vi "tiempo_real.vi"() -> ()   [LabVIEW 2011]
uses:
  <vilib>/Simulation/Scripting/Companion Diagram/SimConfigNode/SimParams.ctl
  <vilib>/Simulation/Scripting/Companion Diagram/SimConfigNode/_simSolvers.ctl
  <vilib>/Simulation/Implementation/Shared/SIMSCR Execution Mode.ctl
  <vilib>/Simulation/Param Hierarchy/Typedefs/SIMPH Param Control Actions.ctl
  <vilib>/Simulation/Implementation/Shared/NILVSim_FinalizeModel.vi
  <vilib>/Simulation/DiscreteLinear/Implementation/NILVSim Discrete Transfer Function Direct.llb/SIM Discrete Transfer Function Direct (SISO CD).vi
  <vilib>/Simulation/DiscreteLinear/Implementation/NILVSim Discrete ZOH.llb/SIM Discrete ZOH (scalar).vi
  <vilib>/Simulation/Nonlinear/Implementation/NILVSim Saturation.llb/SIM Saturation (scalar).vi
  <vilib>/Simulation/SignalDisplay/Implementation/NILVSim Time Waveform.llb/SIM Time Waveform (vector).vi
  <vilib>/Simulation/SignalDisplay/Implementation/NILVSim Time Waveform.llb/SIM Time Waveform (scalar).vi
  <vilib>/Simulation/Implementation/Shared/NILVSim_Manager.vi
  <vilib>/Simulation/Implementation/Shared/NILVSim_ParamChanged.vi
  <vilib>/Simulation/Utility/Implementation/NILVSim Get Time and IsAcceptedStep.vi
  <vilib>/addons/Control Design/_Model Construction/Model Creation.llb/Model Creation SubVI/cd_Create Transfer Function Model.vi
  <vilib>/addons/Control Design/_Utility/Model Viewer.llb/Model Viewer SubVI/cd_Draw Transfer Function Equation (TF).vi
  <vilib>/Simulation/Implementation/Shared/SIM Unbundle Sim Info.vi
  <vilib>/Simulation/Implementation/Shared/NILVSim_GetModelError.vi
  <vilib>/Simulation/Implementation/Shared/SIM Bundle Sim Info.vi
  <vilib>/Simulation/Implementation/Shared/NILVSim_Initialize.vi
  <vilib>/Simulation/Scripting/Companion Diagram/SimConfigNode/SimDog.xnode
  <vilib>/Simulation/Implementation/XNodeFramework/SimXNode/SimX.xnode
  <vilib>/addons/Control Design/_Model Construction/Model Typedefs.llb/CD Transfer Function Model (MIMO).ctl
  <vilib>/addons/Control Design/_Model Construction/Model Typedefs.llb/CD General Elements.ctl
  <vilib>/addons/Control Design/_Model Construction/Model Typedefs.llb/CD Transfer Function Model (SISO).ctl
  <vilib>/addons/Control Design/_Utility/NI_CD_Model Viewer.lvlib
  <vilib>/addons/Control Design/_Model Construction/NI_LinSys_Model Creation.lvlib
  <vilib>/addons/Control Design/_Model Construction/NI_LinSys_Model Typedefs.lvlib
  <vilib>/Simulation/Implementation/Shared/NI_SIM_Implementation.lvlib
panel:
  out "D(z)":picture
  out "?":waveform(dbl)(graph)={"t0"=timestamp(0 s since 1904-01-01), "dt"=1.0, "Y"=[0.0]}
  out "?":waveform(dbl)[](graph)=[{"t0"=timestamp(0 s since 1904-01-01), "dt"=1.0, "Y"=[4.028870584284064]}, {"t0"=timestamp(0 s since 1904-01-01), "dt"=1.0, "Y"=[4.030612244897959]}]
  in  "T":dbl=0.03
  in  "Set Point":dbl(slide)=4.030612244897959 scale=0.0..5.0
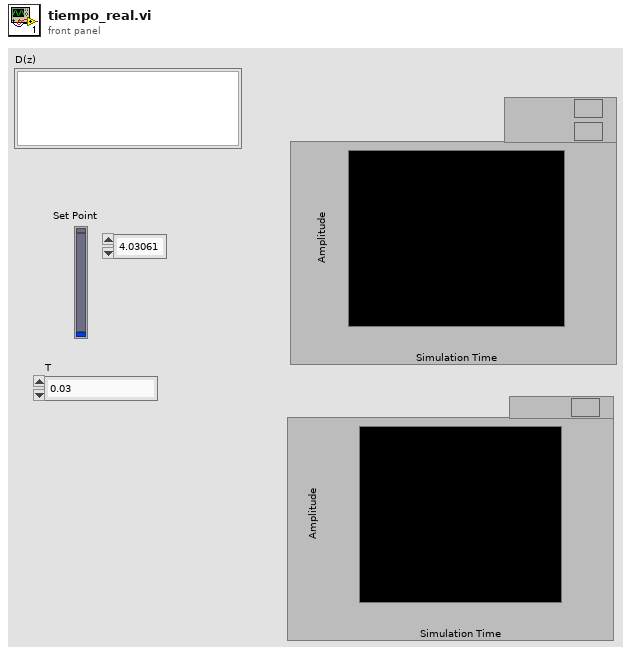
[diagram p1: front panel]
types:
  T1 = typedef "NI_LinSys_Model Typedefs.lvlib/CD Transfer Function Model (MIMO).ctl" = cluster{"properties":T2, "transfer function(s)":T3[][]}
  T2 = typedef "NI_LinSys_Model Typedefs.lvlib/CD General Elements.ctl" = cluster{"Model name":string, "Input names":string[], "Output names":string[], "Input Delays":dbl[], "Output Delays":dbl[], "Sampling Time":dbl, "Notes":string}
  T3 = typedef "NI_LinSys_Model Typedefs.lvlib/CD Transfer Function Model (SISO).ctl" = cluster{"Numerator":dbl[], "Denominator":dbl[], "delay":dbl}
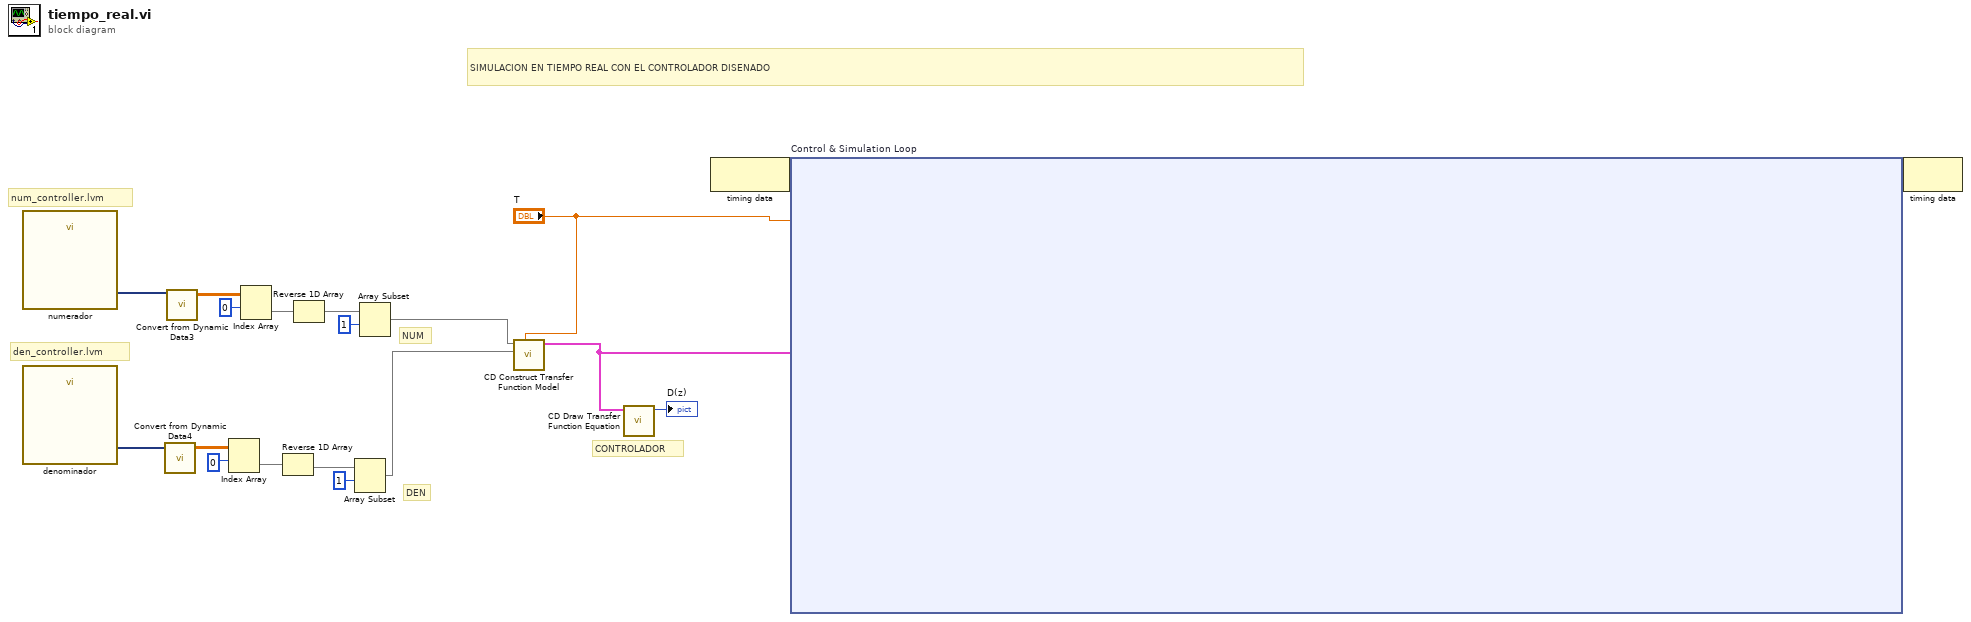
[diagram p0: block diagram]
diagram:
  # "SIMULACION EN TIEMPO REAL CON EL CONTROLADOR DISENADO"
  # "DEN"
  # "NUM"
  # "den_controller.lvm"
  # "num_controller.lvm"
  # "CONTROLADOR"
  n1 = call "numerador"() -> ("Signals"=w4:dynamicdata)  [unwired: 6 in, 5 out]
  n2 = call "denominador"() -> ("Signals"=w3:dynamicdata)  [unwired: 6 in, 5 out]
  n3 = call "Convert from Dynamic Data4"("Dynamic Data Type"=w3) -> ("Array"=w6:dbl[][])  [unwired: 3 in]
  n4 = call "Convert from Dynamic Data3"("Dynamic Data Type"=w4) -> ("Array"=w13:dbl[][])  [unwired: 3 in]
  n5 = Index Array(array=w6, index (row)=0) -> (element=w7:dbl[])  [unwired: 1 in]
  n6 = Index Array(array=w13, index (row)=0) -> (element=w12:dbl[])  [unwired: 1 in]
  n7 = Reverse 1D Array(array=w7) -> (reversed array=w8:dbl[])
  n8 = Reverse 1D Array(array=w12) -> (reversed array=w11:dbl[])
  n9 = Array Subset(array=w8, index=1) -> (w1:dbl[])  [unwired: 1 in]
  n10 = Array Subset(array=w11, index=1) -> (w2:dbl[])  [unwired: 1 in]
  n11 = call-poly <vilib>:"CD Construct Transfer Function Model.vi"("Sampling Time (s)"="T", "Denominator"=w1, "Numerator"=w2) -> ("Transfer Function Model"=w16:T1)  [unwired: 7 in, 1 out]
  n12 = call-poly <vilib>:"CD Draw Transfer Function Equation.vi"("Transfer Function Model"=w16) -> ("Equation"=→"D(z)":picture)  [unwired: 8 in, 2 out]
  n13 = node-c288() -> (w19:variant)  [unwired: 1 in]
  n14 = node-c254 "Control & Simulation Loop"(w19, "T", w16) -> (w18:variant)
  n15 = node-c288(w18) -> ()  [unwired: 1 out]
